vi "rszvl_core_global.vi"() -> ()   [LabVIEW 2014] (continued)
"Command"="DWEL"}]}, {"Name"="rszvl_rngNWASegmentRBW", "Type"=0, "Min?"=TRUE, "Max?"=TRUE, "Entries"=[{"Name"="", "Discrete or Min"=1e-06, "Max"=5000000.0, "Coerced"=0.0, "Command"=""}]}, {"Name"="rszvl_rngNWASegmentSelectivity", "Type"=2, "Min?"=FALSE, "Max?"=FALSE, "Entries"=[{"Name"="RSZVL_VAL_SEG_SELECTIVITY_NORMAL", "Discrete or Min"=0.0, "Max"=0.0, "Coerced"=0.0, "Command"="NORM"}, {"Name"="RSZVL_VAL_SEG_SELECTIVITY_FAST", "Discrete or Min"=1.0, "Max"=0.0, "Coerced"=0.0, "Command"="FAST"}]}, {"Name"="rszvl_rngNWASegmentSweepTime", "Type"=0, "Min?"=TRUE, "Max?"=TRUE, "Entries"=[{"Name"="", "Discrete or Min"=0.0, "Max"=1000.0, "Coerced"=0.0, "Command"=""}]}, {"Name"="rszvl_rngNWASegmentMeasDelay", "Type"=0, "Min?"=TRUE, "Max?"=TRUE, "Entries"=[{"Name"="", "Discrete or Min"=0.0, "Max"=2500.0, "Coerced"=0.0, "Command"=""}]}, {"Name"="rszvl_rngNWASegmentSweepPoints", "Type"=0, "Min?"=TRUE, "Max?"=TRUE, "Entries"=[{"Name"="", "Discrete or Min"=1.0, "Max"=4001.0, "Coerced"=0.0, "Command"=""}]}, {"Name"="rszvl_rngNWAConnectorType", "Type"=2, "Min?"=FALSE, "Max?"=FALSE, "Entries"=[{"Name"="RSZVL_VAL_CONN_N50FEMALE", "Discrete or Min"=0.0, "Max"=0.0, "Coerced"=0.0, "Command"="N50FEMALE"}, {"Name"="RSZVL_VAL_CONN_N50MALE", "Discrete or Min"=1.0, "Max"=0.0, "Coerced"=0.0, "Command"="N50MALE"}, {"Name"="RSZVL_VAL_CONN_N75FEMALE", "Discrete or Min"=2.0, "Max"=0.0, "Coerced"=0.0, "Command"="N75FEMALE"}, {"Name"="RSZVL_VAL_CONN_N75MALE", "Discrete or Min"=3.0, "Max"=0.0, "Coerced"=0.0, "Command"="N75MALE"}, {"Name"="RSZVL_VAL_CONN_PC7", "Discrete or Min"=4.0, "Max"=0.0, "Coerced"=0.0, "Command"="PC7"}, {"Name"="RSZVL_VAL_CONN_PC35FEMALE", "Discrete or Min"=5.0, "Max"=0.0, "Coerced"=0.0, "Command"="PC35FEMALE"}, {"Name"="RSZVL_VAL_CONN_PC35MALE", "Discrete or Min"=6.0, "Max"=0.0, "Coerced"=0.0, "Command"="PC35MALE"}, {"Name"="RSZVL_VAL_CONN_PC292FEMALE", "Discrete or Min"=7.0, "Max"=0.0, "Coerced"=0.0, "Command"="PC292FEMALE"}, {"Name"="RSZVL_VAL_CONN_PC292MALE", "Discrete or Min"=8.0, "Max"=0.0, "Coerced"=0.0, "Command"="PC292MALE"}, {"Name"="RSZVL_VAL_CONN_UFEMALE1", "Discrete or Min"=9.0, "Max"=0.0, "Coerced"=0.0, "Command"="UFEMALE1"}, {"Name"="RSZVL_VAL_CONN_UMALE1", "Discrete or Min"=10.0, "Max"=0.0, "Coerced"=0.0, "Command"="UMALE1"}, {"Name"="RSZVL_VAL_CONN_UFEMALE2", "Discrete or Min"=11.0, "Max"=0.0, "Coerced"=0.0, "Command"="UFEMALE2"}, {"Name"="RSZVL_VAL_CONN_UMALE2", "Discrete or Min"=12.0, "Max"=0.0, "Coerced"=0.0, "Command"="UMALE2"}]}, {"Name"="rszvl_rngNWASameConnectorsAtPorts", "Type"=2, "Min?"=FALSE, "Max?"=FALSE, "Entries"=[{"Name"="RSZVL_VAL_CONN_PORTS_SINGLE", "Discrete or Min"=0.0, "Max"=0.0, "Coerced"=0.0, "Command"="SING"}, {"Name"="RSZVL_VAL_CONN_PORTS_ALL", "Discrete or Min"=1.0, "Max"=0.0, "Coerced"=0.0, "Command"="ALL"}]}, {"Name"="rszvl_rngNWAOffsetLoss", "Type"=0, "Min?"=TRUE, "Max?"=TRUE, "Entries"=[{"Name"="", "Discrete or Min"=-200.0, "Max"=200.0, "Coerced"=0.0, "Command"=""}]}, {"Name"="rszvl_rngNWASourcePower", "Type"=0, "Min?"=TRUE, "Max?"=TRUE, "Entries"=[{"Name"="", "Discrete or Min"=-300.0, "Max"=20.0, "Coerced"=0.0, "Command"=""}]}, {"Name"="rszvl_rngNWATraceXOffset", "Type"=0, "Min?"=TRUE, "Max?"=TRUE, "Entries"=[{"Name"="", "Discrete or Min"=-999000000000.0, "Max"=999000000000.0, "Coerced"=0.0, "Command"=""}]}, {"Name"="rszvl_rngNWATraceFormat", "Type"=2, "Min?"=FALSE, "Max?"=FALSE, "Entries"=[{"Name"="RSZVL_VAL_TRAC_FORM_MLIN", "Discrete or Min"=0.0, "Max"=0.0, "Coerced"=0.0, "Command"="MLIN"}, {"Name"="RSZVL_VAL_TRAC_FORM_MLOG", "Discrete or Min"=1.0, "Max"=0.0, "Coerced"=0.0, "Command"="MLOG"}, {"Name"="RSZVL_VAL_TRAC_FORM_PHAS", "Discrete or Min"=2.0, "Max"=0.0, "Coerced"=0.0, "Command"="PHAS"}, {"Name"="RSZVL_VAL_TRAC_FORM_UPH", "Discrete or Min"=3.0, "Max"=0.0, "Coerced"=0.0, "Command"="UPH"}, {"Name"="RSZVL_VAL_TRAC_FORM_POL", "Discrete or Min"=4.0, "Max"=0.0, "Coerced"=0.0, "Command"="POL"}, {"Name"="RSZVL_VAL_TRAC_FORM_SMIT", "Discrete or Min"=5.0, "Max"=0.0, "Coerced"=0.0, "Command"="SMIT"}, {"Name"="RSZVL_VAL_TRAC_FORM_ISM", "Discrete or Min"=6.0, "Max"=0.0, "Coerced"=0.0, "Command"="ISM"}, {"Name"="RSZVL_VAL_TRAC_FORM_GDEL", "Discrete or Min"=7.0, "Max"=0.0, "Coerced"=0.0, "Command"="GDEL"}, {"Name"="RSZVL_VAL_TRAC_FORM_REAL", "Discrete or Min"=8.0, "Max"=0.0, "Coerced"=0.0, "Command"="REAL"}, {"Name"="RSZVL_VAL_TRAC_FORM_IMAG", "Discrete or Min"=9.0, "Max"=0.0, "Coerced"=0.0, "Command"="IMAG"}, {"Name"="RSZVL_VAL_TRAC_FORM_SWR", "Discrete or Min"=10.0, "Max"=0.0, "Coerced"=0.0, "Command"="SWR"}]}, {"Name"="rszvl_rngNWATraceMathFunction", "Type"=2, "Min?"=FALSE, "Max?"=FALSE, "Entries"=[{"Name"="RSZVL_VAL_TRAC_MATH_FUNC_NORM", "Discrete or Min"=0.0, "Max"=0.0, "Coerced"=0.0, "Command"="NORM"}, {"Name"="RSZVL_VAL_TRAC_MATH_FUNC_SUBT", "Discrete or Min"=1.0, "Max"=0.0, "Coerced"=0.0, "Command"="SUBT"}, {"Name"="RSZVL_VAL_TRAC_MATH_FUNC_DIV", "Discrete or Min"=2.0, "Max"=0.0, "Coerced"=0.0, "Command"="DIV"}]}, {"Name"="rszvl_rngNWATraceSmoothing", "Type"=0, "Min?"=TRUE, "Max?"=TRUE, "Entries"=[{"Name"="", "Discrete or Min"=0.05, "Max"=100.0, "Coerced"=0.0, "Command"=""}]}, {"Name"="rszvl_rngNWATraceMaxHold", "Type"=2, "Min?"=FALSE, "Max?"=FALSE, "Entries"=[{"Name"="RSZVL_VAL_TRAC_PHOL_OFF", "Discrete or Min"=0.0, "Max"=0.0, "Coerced"=0.0, "Command"="OFF"}, {"Name"="RSZVL_VAL_TRAC_PHOL_MAX", "Discrete or Min"=1.0, "Max"=0.0, "Coerced"=0.0, "Command"="MAX"}]}, {"Name"="rszvl_rngNWADeleteMemTrace", "Type"=2, "Min?"=FALSE, "Max?"=FALSE, "Entries"=[{"Name"="RSZVL_VAL_TRAC_DELETE_MDAT1", "Discrete or Min"=0.0, "Max"=0.0, "Coerced"=0.0, "Command"="MDATA1"}, {"Name"="RSZVL_VAL_TRAC_DELETE_MDAT2", "Discrete or Min"=1.0, "Max"=0.0, "Coerced"=0.0, "Command"="MDATA2"}, {"Name"="RSZVL_VAL_TRAC_DELETE_MDAT3", "Discrete or Min"=2.0, "Max"=0.0, "Coerced"=0.0, "Command"="MDATA3"}, {"Name"="RSZVL_VAL_TRAC_DELETE_MDAT4", "Discrete or Min"=3.0, "Max"=0.0, "Coerced"=0.0, "Command"="MDATA4"}, {"Name"="RSZVL_VAL_TRAC_DELETE_MDAT5", "Discrete or Min"=4.0, "Max"=0.0, "Coerced"=0.0, "Command"="MDATA5"}, {"Name"="RSZVL_VAL_TRAC_DELETE_MDAT6", "Discrete or Min"=5.0, "Max"=0.0, "Coerced"=0.0, "Command"="MDATA6"}, {"Name"="RSZVL_VAL_TRAC_DELETE_MDAT7", "Discrete or Min"=6.0, "Max"=0.0, "Coerced"=0.0, "Command"="MDATA7"}, {"Name"="RSZVL_VAL_TRAC_DELETE_MDAT8", "Discrete or Min"=7.0, "Max"=0.0, "Coerced"=0.0, "Command"="MDATA8"}]}, {"Name"="rszvl_rngNWATraceEvalRange", "Type"=2, "Min?"=FALSE, "Max?"=FALSE, "Entries"=[{"Name"="RSZVL_VAL_TRAC_EVAL_FULL_SPAN", "Discrete or Min"=0.0, "Max"=0.0, "Coerced"=0.0, "Command"="0"}, {"Name"="RSZVL_VAL_TRAC_EVAL_1", "Discrete or Min"=1.0, "Max"=0.0, "Coerced"=0.0, "Command"="1"}, {"Name"="RSZVL_VAL_TRAC_EVAL_2", "Discrete or Min"=2.0, "Max"=0.0, "Coerced"=0.0, "Command"="2"}, {"Name"="RSZVL_VAL_TRAC_EVAL_3", "Discrete or Min"=3.0, "Max"=0.0, "Coerced"=0.0, "Command"="3"}, {"Name"="RSZVL_VAL_TRAC_EVAL_4", "Discrete or Min"=4.0, "Max"=0.0, "Coerced"=0.0, "Command"="4"}, {"Name"="RSZVL_VAL_TRAC_EVAL_5", "Discrete or Min"=5.0, "Max"=0.0, "Coerced"=0.0, "Command"="5"}, {"Name"="RSZVL_VAL_TRAC_EVAL_6", "Discrete or Min"=6.0, "Max"=0.0, "Coerced"=0.0, "Command"="6"}, {"Name"="RSZVL_VAL_TRAC_EVAL_7", "Discrete or Min"=7.0, "Max"=0.0, "Coerced"=0.0, "Command"="7"}, {"Name"="RSZVL_VAL_TRAC_EVAL_8", "Discrete or Min"=8.0, "Max"=0.0, "Coerced"=0.0, "Command"="8"}, {"Name"="RSZVL_VAL_TRAC_EVAL_9", "Discrete or Min"=9.0, "Max"=0.0, "Coerced"=0.0, "Command"="9"}, {"Name"="RSZVL_VAL_TRAC_EVAL_10", "Discrete or Min"=10.0, "Max"=0.0, "Coerced"=0.0, "Command"="10"}]}, {"Name"="rszvl_rngNWATraceEvalRangeStart", "Type"=0, "Min?"=TRUE, "Max?"=TRUE, "Entries"=[{"Name"="", "Discrete or Min"=-1000000000000.0, "Max"=999999999999.0, "Coerced"=0.0, "Command"=""}]}, {"Name"="rszvl_rngNWATraceEvalRangeStop", "Type"=0, "Min?"=TRUE, "Max?"=TRUE, "Entries"=[{"Name"="", "Discrete or Min"=-999999999999.0, "Max"=1000000000000.0, "Coerced"=0.0, "Command"=""}]}, {"Name"="rszvl_rngNWAMarkerStimulus", "Type"=0, "Min?"=TRUE, "Max?"=TRUE, "Entries"=[{"Name"="", "Discrete or Min"=-990000000000.0, "Max"=990000000000.0, "Coerced"=0.0, "Command"=""}]}, {"Name"="rszvl_rngNWAMarkerMode", "Type"=2, "Min?"=FALSE, "Max?"=FALSE, "Entries"=[{"Name"="RSZVL_VAL_MARK_MODE_CONT", "Discrete or Min"=0.0, "Max"=0.0, "Coerced"=0.0, "Command"="CONT"}, {"Name"="RSZVL_VAL_MARK_MODE_DISC", "Discrete or Min"=1.0, "Max"=0.0, "Coerced"=0.0, "Command"="DISC"}]}, {"Name"="rszvl_rngNWAMarkerType", "Type"=2, "Min?"=FALSE, "Max?"=FALSE, "Entries"=[{"Name"="RSZVL_VAL_MARKER_TYPE_NORM", "Discrete or Min"=0.0, "Max"=0.0, "Coerced"=0.0, "Command"="NORM"}, {"Name"="RSZVL_VAL_MARKER_TYPE_FIX", "Discrete or Min"=1.0, "Max"=0.0, "Coerced"=0.0, "Command"="FIX"}]}, {"Name"="rszvl_rngNWAMarkerFormat", "Type"=2, "Min?"=FALSE, "Max?"=FALSE, "Entries"=[{"Name"="RSZVL_VAL_MARK_FORM_MLIN", "Discrete or Min"=0.0, "Max"=0.0, "Coerced"=0.0, "Command"="MLIN"}, {"Name"="RSZVL_VAL_MARK_FORM_MLOG", "Discrete or Min"=1.0, "Max"=0.0, "Coerced"=0.0, "Command"="MLOG"}, {"Name"="RSZVL_VAL_MARK_FORM_PHAS", "Discrete or Min"=2.0, "Max"=0.0, "Coerced"=0.0, "Command"="PHAS"}, {"Name"="RSZVL_VAL_MARK_FORM_POL", "Discrete or Min"=3.0, "Max"=0.0, "Coerced"=0.0, "Command"="POL"}, {"Name"="RSZVL_VAL_MARK_FORM_GDEL", "Discrete or Min"=4.0, "Max"=0.0, "Coerced"=0.0, "Command"="GDEL"}, {"Name"="RSZVL_VAL_MARK_FORM_REAL", "Discrete or Min"=5.0, "Max"=0.0, "Coerced"=0.0, "Command"="REAL"}, {"Name"="RSZVL_VAL_MARK_FORM_IMAG", "Discrete or Min"=6.0, "Max"=0.0, "Coerced"=0.0, "Command"="IMAG"}, {"Name"="RSZVL_VAL_MARK_FORM_SWR", "Discrete or Min"=7.0, "Max"=0.0, "Coerced"=0.0, "Command"="SWR"}, {"Name"="RSZVL_VAL_MARK_FORM_LINP", "Discrete or Min"=8.0, "Max"=0.0, "Coerced"=0.0, "Command"="LINP"}, {"Name"="RSZVL_VAL_MARK_FORM_LOGP", "Discrete or Min"=9.0, "Max"=0.0, "Coerced"=0.0, "Command"="LOGP"}, {"Name"="RSZVL_VAL_MARK_FORM_IMP", "Discrete or Min"=10.0, "Max"=0.0, "Coerced"=0.0, "Command"="IMP"}, {"Name"="RSZVL_VAL_MARK_FORM_ADM", "Discrete or Min"=11.0, "Max"=0.0, "Coerced"=0.0, "Command"="ADM"}]}, {"Name"="rszvl_rngNWAMarkerSearch", "Type"=2, "Min?"=FALSE, "Max?"=FALSE, "Entries"=[{"Name"="RSZVL_VAL_MARK_SEARCH_MAX", "Discrete or Min"=0.0, "Max"=0.0, "Coerced"=0.0, "Command"="MAX"}, {"Name"="RSZVL_VAL_MARK_SEARCH_MIN", "Discrete or Min"=1.0, "Max"=0.0, "Coerced"=0.0, "Command"="MIN"}, {"Name"="RSZVL_VAL_MARK_SEARCH_RPE", "Discrete or Min"=2.0, "Max"=0.0, "Coerced"=0.0, "Command"="RPE"}, {"Name"="RSZVL_VAL_MARK_SEARCH_LPE", "Discrete or Min"=3.0, "Max"=0.0, "Coerced"=0.0, "Command"="LPE"}, {"Name"="RSZVL_VAL_MARK_SEARCH_NPE", "Discrete or Min"=4.0, "Max"=0.0, "Coerced"=0.0, "Command"="NPE"}, {"Name"="RSZVL_VAL_MARK_SEARCH_TARG", "Discrete or Min"=5.0, "Max"=0.0, "Coerced"=0.0, "Command"="TARG"}, {"Name"="RSZVL_VAL_MARK_SEARCH_LTAR", "Discrete or Min"=6.0, "Max"=0.0, "Coerced"=0.0, "Command"="LTAR"}, {"Name"="RSZVL_VAL_MARK_SEARCH_RTAR", "Discrete or Min"=7.0, "Max"=0.0, "Coerced"=0.0, "Command"="RTAR"}, {"Name"="RSZVL_VAL_MARK_SEARCH_BFIL", "Discrete or Min"=8.0, "Max"=0.0, "Coerced"=0.0, "Command"="BFIL"}]}, {"Name"="rszvl_rngNWAMarkerBFilterSearchMode", "Type"=2, "Min?"=FALSE, "Max?"=FALSE, "Entries"=[{"Name"="RSZVL_VAL_MARK_BFIL_SEARCH_BPAS", "Discrete or Min"=0.0, "Max"=0.0, "Coerced"=0.0, "Command"="BPAS"}, {"Name"="RSZVL_VAL_MARK_BFIL_SEARCH_BST", "Discrete or Min"=1.0, "Max"=0.0, "Coerced"=0.0, "Command"="BST"}, {"Name"="RSZVL_VAL_MARK_BFIL_SEARCH_BPRM", "Discrete or Min"=2.0, "Max"=0.0, "Coerced"=0.0, "Command"="BPRM"}, {"Name"="RSZVL_VAL_MARK_BFIL_SEARCH_BSRM", "Discrete or Min"=3.0, "Max"=0.0, "Coerced"=0.0, "Command"="BSRM"}]}, {"Name"="rszvl_rngNWAMarkerSearchRange", "Type"=2, "Min?"=FALSE, "Max?"=FALSE, "Entries"=[{"Name"="RSZVL_VAL_MARK_FULL_SPAN", "Discrete or Min"=0.0, "Max"=0.0, "Coerced"=0.0, "Command"="0"}, {"Name"="RSZVL_VAL_MARK_RANGE_1", "Discrete or Min"=1.0, "Max"=0.0, "Coerced"=0.0, "Command"="1"}, {"Name"="RSZVL_VAL_MARK_RANGE_2", "Discrete or Min"=2.0, "Max"=0.0, "Coerced"=0.0, "Command"="2"}, {"Name"="RSZVL_VAL_MARK_RANGE_3", "Discrete or Min"=3.0, "Max"=0.0, "Coerced"=0.0, "Command"="3"}, {"Name"="RSZVL_VAL_MARK_RANGE_4", "Discrete or Min"=4.0, "Max"=0.0, "Coerced"=0.0, "Command"="4"}, {"Name"="RSZVL_VAL_MARK_RANGE_5", "Discrete or Min"=5.0, "Max"=0.0, "Coerced"=0.0, "Command"="5"}, {"Name"="RSZVL_VAL_MARK_RANGE_6", "Discrete or Min"=6.0, "Max"=0.0, "Coerced"=0.0, "Command"="6"}, {"Name"="RSZVL_VAL_MARK_RANGE_7", "Discrete or Min"=7.0, "Max"=0.0, "Coerced"=0.0, "Command"="7"}, {"Name"="RSZVL_VAL_MARK_RANGE_8", "Discrete or Min"=8.0, "Max"=0.0, "Coerced"=0.0, "Command"="8"}, {"Name"="RSZVL_VAL_MARK_RANGE_9", "Discrete or Min"=9.0, "Max"=0.0, "Coerced"=0.0, "Command"="9"}, {"Name"="RSZVL_VAL_MARK_RANGE_10", "Discrete or Min"=10.0, "Max"=0.0, "Coerced"=0.0, "Command"="10"}]}, {"Name"="rszvl_rngNWALimitRDOMComplex", "Type"=2, "Min?"=FALSE, "Max?"=FALSE, "Entries"=[{"Name"="RSZVL_VAL_LIM_RDOM_COMP_S", "Discrete or Min"=0.0, "Max"=0.0, "Coerced"=0.0, "Command"="S"}, {"Name"="RSZVL_VAL_LIM_RDOM_COMP_SINV", "Discrete or Min"=1.0, "Max"=0.0, "Coerced"=0.0, "Command"="SINV"}, {"Name"="RSZVL_VAL_LIM_RDOM_COMP_Y", "Discrete or Min"=2.0, "Max"=0.0, "Coerced"=0.0, "Command"="Y"}, {"Name"="RSZVL_VAL_LIM_RDOM_COMP_Z", "Discrete or Min"=3.0, "Max"=0.0, "Coerced"=0.0, "Command"="Z"}, {"Name"="RSZVL_VAL_LIM_RDOM_COMP_YREL", "Discrete or Min"=4.0, "Max"=0.0, "Coerced"=0.0, "Command"="YREL"}, {"Name"="RSZVL_VAL_LIM_RDOM_COMP_ZREL", "Discrete or Min"=5.0, "Max"=0.0, "Coerced"=0.0, "Command"="ZREL"}]}, {"Name"="rszvl_rngNWALimitRDOMFormat", "Type"=2, "Min?"=FALSE, "Max?"=FALSE, "Entries"=[{"Name"="RSZVL_VAL_LIM_RDOM_FORM_COMP", "Discrete or Min"=0.0, "Max"=0.0, "Coerced"=0.0, "Command"="COMP"}, {"Name"="RSZVL_VAL_LIM_RDOM_FORM_MAGN", "Discrete or Min"=1.0, "Max"=0.0, "Coerced"=0.0, "Command"="MAGN"}, {"Name"="RSZVL_VAL_LIM_RDOM_FORM_PHAS", "Discrete or Min"=2.0, "Max"=0.0, "Coerced"=0.0, "Command"="PHAS"}, {"Name"="RSZVL_VAL_LIM_RDOM_FORM_REAL", "Discrete or Min"=3.0, "Max"=0.0, "Coerced"=0.0, "Command"="REAL"}, {"Name"="RSZVL_VAL_LIM_RDOM_FORM_IMAG", "Discrete or Min"=4.0, "Max"=0.0, "Coerced"=0.0, "Command"="IMAG"}, {"Name"="RSZVL_VAL_LIM_RDOM_FORM_SWR", "Discrete or Min"=5.0, "Max"=0.0, "Coerced"=0.0, "Command"="SWR"}, {"Name"="RSZVL_VAL_LIM_RDOM_FORM_GDEL", "Discrete or Min"=6.0, "Max"=0.0, "Coerced"=0.0, "Command"="GDEL"}, {"Name"="RSZVL_VAL_LIM_RDOM_FORM_L", "Discrete or Min"=7.0, "Max"=0.0, "Coerced"=0.0, "Command"="L"}, {"Name"="RSZVL_VAL_LIM_RDOM_FORM_C", "Discrete or Min"=8.0, "Max"=0.0, "Coerced"=0.0, "Command"="C"}]}, {"Name"="rszvl_rngNWALimitRDOMSpacing", "Type"=2, "Min?"=FALSE, "Max?"=FALSE, "Entries"=[{"Name"="RSZVL_VAL_LIM_RDOM_SPAC_LIN", "Discrete or Min"=0.0, "Max"=0.0, "Coerced"=0.0, "Command"="LIN"}, {"Name"="RSZVL_VAL_LIM_RDOM_SPAC_LOG", "Discrete or Min"=1.0, "Max"=0.0, "Coerced"=0.0, "Command"="LOG"}, {"Name"="RSZVL_VAL_LIM_RDOM_SPAC_DB", "Discrete or Min"=2.0, "Max"=0.0, "Coerced"=0.0, "Command"="DB"}, {"Name"="RSZVL_VAL_LIM_RDOM_SPAC_SIC", "Discrete or Min"=3.0, "Max"=0.0, "Coerced"=0.0, "Command"="SIC"}]}, {"Name"="rszvl_rngNWALimitSegmType", "Type"=2, "Min?"=FALSE, "Max?"=FALSE, "Entries"=[{"Name"="RSZVL_VAL_LIMIT_OFF", "Discrete or Min"=0.0, "Max"=0.0, "Coerced"=0.0, "Command"="OFF"}, {"Name"="RSZVL_VAL_LIMIT_UPPER", "Discrete or Min"=1.0, "Max"=0.0, "Coerced"=0.0, "Command"="LMAX"}, {"Name"="RSZVL_VAL_LIMIT_LOWER", "Discrete or Min"=2.0, "Max"=0.0, "Coerced"=0.0, "Command"="LMIN"}]}, {"Name"="rszvl_rngNWAParamConversion", "Type"=2, "Min?"=FALSE, "Max?"=FALSE, "Entries"=[{"Name"="RSZVL_VAL_CONV_S", "Discrete or Min"=0.0, "Max"=0.0, "Coerced"=0.0, "Command"="S"}, {"Name"="RSZVL_VAL_CONV_Y", "Discrete or Min"=1.0, "Max"=0.0, "Coerced"=0.0, "Command"="Y"}, {"Name"="RSZVL_VAL_CONV_Z", "Discrete or Min"=2.0, "Max"=0.0, "Coerced"=0.0, "Command"="Z"}]}, {"Name"="rszvl_rngNWAColorScheme", "Type"=2, "Min?"=FALSE, "Max?"=FALSE, "Entries"=[{"Name"="RSZVL_VAL_COLOR_DBACKGROUND", "Discrete or Min"=0.0, "Max"=0.0, "Coerced"=0.0, "Command"="DBAC"}, {"Name"="RSZVL_VAL_COLOR_LBACKGROUND", "Discrete or Min"=1.0, "Max"=0.0, "Coerced"=0.0, "Command"="LBAC"}, {"Name"="RSZVL_VAL_COLOR_BW_LSTYLES", "Discrete or Min"=2.0, "Max"=0.0, "Coerced"=0.0, "Command"="BWLS"}, {"Name"="RSZVL_VAL_COLOR_BW_SOLID", "Discrete or Min"=3.0, "Max"=0.0, "Coerced"=0.0, "Command"="BWS"}]}, {"Name"="rszvl_rngNWAPresetScope", "Type"=2, "Min?"=FALSE, "Max?"=FALSE, "Entries"=[{"Name"="RSZVL_VAL_PRESET_SINGLE", "Discrete or Min"=0.0, "Max"=0.0, "Coerced"=0.0, "Command"="SING"}, {"Name"="RSZVL_VAL_PRESET_ALL", "Discrete or Min"=1.0, "Max"=0.0, "Coerced"=0.0, "Command"="ALL"}]}, {"Name"="rszvl_rngInstrMode", "Type"=2, "Min?"=FALSE, "Max?"=FALSE, "Entries"=[{"Name"="RSZVL_VAL_SAN", "Discrete or Min"=0.0, "Max"=0.0, "Coerced"=0.0, "Command"="SAN"}, {"Name"="RSZVL_VAL_NWA", "Discrete or Min"=1.0, "Max"=0.0, "Coerced"=0.0, "Command"="NWA"}, {"Name"="RSZVL_VAL_NOISE", "Discrete or Min"=2.0, "Max"=0.0, "Coerced"=0.0, "Command"="NOIS"}, {"Name"="RSZVL_VAL_BWCD", "Discrete or Min"=3.0, "Max"=0.0, "Coerced"=0.0, "Command"="BWCD"}, {"Name"="RSZVL_VAL_WLAN", "Discrete or Min"=4.0, "Max"=0.0, "Coerced"=0.0, "Command"="WLAN"}, {"Name"="RSZVL_VAL_WIMAX", "Discrete or Min"=5.0, "Max"=0.0, "Coerced"=0.0, "Command"="WIM"}, {"Name"="RSZVL_VAL_ADEM", "Discrete or Min"=6.0, "Max"=0.0, "Coerced"=0.0, "Command"="ADEM"}, {"Name"="RSZVL_VAL_BTO", "Discrete or Min"=7.0, "Max"=0.0, "Coerced"=0.0, "Command"="BTO"}, {"Name"="RSZVL_VAL_CATV", "Discrete or Min"=8.0, "Max"=0.0, "Coerced"=0.0, "Command"="CATV"}]}, {"Name"="rszvl_rngNWADFaultStart", "Type"=0, "Min?"=TRUE, "Max?"=TRUE, "Entries"=[{"Name"="", "Discrete or Min"=-5.0, "Max"=9.9999, "Coerced"=0.0, "Command"=""}]}, {"Name"="rszvl_rngNWADFaultStop", "Type"=0, "Min?"=TRUE, "Max?"=TRUE, "Entries"=[{"Name"="", "Discrete or Min"=-4.999, "Max"=10.0, "Coerced"=0.0, "Command"=""}]}, {"Name"="rszvl_rngNWADFaultSpan", "Type"=0, "Min?"=TRUE, "Max?"=TRUE, "Entries"=[{"Name"="", "Discrete or Min"=0.001, "Max"=15.0, "Coerced"=0.0, "Command"=""}]}, {"Name"="rszvl_rngNWASegmentAtten", "Type"=0, "Min?"=TRUE, "Max?"=TRUE, "Entries"=[{"Name"="", "Discrete or Min"=0.0, "Max"=30.0, "Coerced"=0.0, "Command"=""}]}, {"Name"="rszvl_rngNWASegmentPower", "Type"=0, "Min?"=TRUE, "Max?"=TRUE, "Entries"=[{"Name"="", "Discrete or Min"=-40.0, "Max"=10.0, "Coerced"=0.0, "Command"=""}]}, {"Name"="rszvl_rngHcopyPageSettings", "Type"=2, "Min?"=FALSE, "Max?"=FALSE, "Entries"=[{"Name"="RSZVL_VAL_HCOPY_ACT", "Discrete or Min"=0.0, "Max"=0.0, "Coerced"=0.0, "Command"="ACT"}, {"Name"="RSZVL_VAL_HCOPY_ALL", "Discrete or Min"=1.0, "Max"=0.0, "Coerced"=0.0, "Command"="ALL"}, {"Name"="RSZVL_VAL_HCOPY_SING", "Discrete or Min"=2.0, "Max"=0.0, "Coerced"=0.0, "Command"="SING"}]}, {"Name"="rszvl_rngNWAGetCalState", "Type"=2, "Min?"=FALSE, "Max?"=FALSE, "Entries"=[{"Name"="RSZVL_CALSTATE_CAL", "Discrete or Min"=0.0, "Max"=0.0, "Coerced"=0.0, "Command"="CAL"}, {"Name"="RSZVL_CALSTATE_CAI", "Discrete or Min"=1.0, "Max"=0.0, "Coerced"=0.0, "Command"="CAI"}, {"Name"="RSZVL_CALSTATE_CA", "Discrete or Min"=2.0, "Max"=0.0, "Coerced"=0.0, "Command"="CA?"}, {"Name"="RSZVL_CALSTATE_CAV", "Discrete or Min"=3.0, "Max"=0.0, "Coerced"=0.0, "Command"="CAV"}, {"Name"="RSZVL_CALSTATE_CALOFF", "Discrete or Min"=4.0, "Max"=0.0, "Coerced"=0.0, "Command"="CAL OFF"}]}, {"Name"="rszvl_rngFmTriggerSource", "Type"=2, "Min?"=FALSE, "Max?"=FALSE, "Entries"=[{"Name"="RSZVL_VAL_TRG_IMM", "Discrete or Min"=0.0, "Max"=0.0, "Coerced"=0.0, "Command"="IMM"}, {"Name"="RSZVL_VAL_TRG_EXT", "Discrete or Min"=1.0, "Max"=0.0, "Coerced"=0.0, "Command"="EXT"}, {"Name"="RSZVL_VAL_TRG_IFP", "Discrete or Min"=2.0, "Max"=0.0, "Coerced"=0.0, "Command"="IFP"}, {"Name"="RSZVL_VAL_TRG_FM", "Discrete or Min"=3.0, "Max"=0.0, "Coerced"=0.0, "Command"="FM"}, {"Name"="RSZVL_VAL_TRG_AM", "Discrete or Min"=4.0, "Max"=0.0, "Coerced"=0.0, "Command"="AM"}, {"Name"="RSZVL_VAL_TRG_PM", "Discrete or Min"=5.0, "Max"=0.0, "Coerced"=0.0, "Command"="PM"}, {"Name"="RSZVL_VAL_TRG_AMR", "Discrete or Min"=6.0, "Max"=0.0, "Coerced"=0.0, "Command"="AMR"}]}, {"Name"="rszvl_rngAdemTrigAMLevelAbs", "Type"=0, "Min?"=TRUE, "Max?"=TRUE, "Entries"=[{"Name"="", "Discrete or Min"=-100.0, "Max"=30.0, "Coerced"=0.0, "Command"=""}]}, {"Name"="rszvl_rngAdemTrigAMLevelRel", "Type"=0, "Min?"=TRUE, "Max?"=TRUE, "Entries"=[{"Name"="", "Discrete or Min"=-100.0, "Max"=100.0, "Coerced"=0.0, "Command"=""}]}, {"Name"="rszvl_rngAdemTrigFMLevel", "Type"=0, "Min?"=TRUE, "Max?"=TRUE, "Entries"=[{"Name"="", "Discrete or Min"=-10000000.0, "Max"=10000000.0, "Coerced"=0.0, "Command"=""}]}, {"Name"="rszvl_rngAdemTrigPMLevel", "Type"=0, "Min?"=TRUE, "Max?"=TRUE, "Entries"=[{"Name"="", "Discrete or Min"=-1000.0, "Max"=1000.0, "Coerced"=0.0, "Command"=""}]}, {"Name"="rszvl_rngCoupling", "Type"=2, "Min?"=FALSE, "Max?"=FALSE, "Entries"=[{"Name"="RSZVL_VAL_DC", "Discrete or Min"=0.0, "Max"=0.0, "Coerced"=0.0, "Command"="DC"}, {"Name"="RSZVL_VAL_AC", "Discrete or Min"=1.0, "Max"=0.0, "Coerced"=0.0, "Command"="AC"}]}, {"Name"="rszvl_rngFmBwid", "Type"=0, "Min?"=TRUE, "Max?"=TRUE, "Entries"=[{"Name"="", "Discrete or Min"=100.0, "Max"=50000000.0, "Coerced"=0.0, "Command"=""}]}, {"Name"="rszvl_rngAdemPhaseWrap", "Type"=2, "Min?"=FALSE, "Max?"=FALSE, "Entries"=[{"Name"="RSZVL_VAL_ADEM_UPHAS", "Discrete or Min"=0.0, "Max"=0.0, "Coerced"=0.0, "Command"="UPH"}, {"Name"="RSZVL_VAL_ADEM_PHAS", "Discrete or Min"=1.0, "Max"=0.0, "Coerced"=0.0, "Command"="PHAS"}]}, {"Name"="rszvl_rngUnitAngle", "Type"=2, "Min?"=FALSE, "Max?"=FALSE, "Entries"=[{"Name"="RSZVL_VAL_UNIT_ANGLE_DEG", "Discrete or Min"=0.0, "Max"=0.0, "Coerced"=0.0, "Command"="DEG"}, {"Name"="RSZVL_VAL_UNIT_ANGLE_RAD", "Discrete or Min"=1.0, "Max"=0.0, "Coerced"=0.0, "Command"="RAD"}]}, {"Name"="rszvl_rngAdemBandRes", "Type"=0, "Min?"=TRUE, "Max?"=TRUE, "Entries"=[{"Name"="", "Discrete or Min"=1.0, "Max"=10000000.0, "Coerced"=0.0, "Command"=""}]}, {"Name"="rszvl_rngHpasFilterFreq", "Type"=1, "Min?"=FALSE, "Max?"=FALSE, "Entries"=[{"Name"="", "Discrete or Min"=0.0, "Max"=0.0, "Coerced"=50.0, "Command"=""}, {"Name"="", "Discrete or Min"=0.0, "Max"=0.0, "Coerced"=300.0, "Command"=""}]}, {"Name"="rszvl_rngLpasFiltFreq", "Type"=1, "Min?"=FALSE, "Max?"=FALSE, "Entries"=[{"Name"="", "Discrete or Min"=0.0, "Max"=0.0, "Coerced"=3000.0, "Command"=""}, {"Name"="", "Discrete or Min"=0.0, "Max"=0.0, "Coerced"=15000.0, "Command"=""}, {"Name"="", "Discrete or Min"=0.0, "Max"=0.0, "Coerced"=150000.0, "Command"=""}]}, {"Name"="rszvl_rngFiltDempTimeConst", "Type"=1, "Min?"=FALSE, "Max?"=FALSE, "Entries"=[{"Name"="", "Discrete or Min"=0.0, "Max"=0.0, "Coerced"=2.5e-05, "Command"=""}, {"Name"="", "Discrete or Min"=0.0, "Max"=0.0, "Coerced"=5e-05, "Command"=""}, {"Name"="", "Discrete or Min"=0.0, "Max"=0.0, "Coerced"=7.5e-05, "Command"=""}, {"Name"="", "Discrete or Min"=0.0, "Max"=0.0, "Coerced"=0.00075, "Command"=""}]}, {"Name"="rszvl_rngFiltDempPctConst", "Type"=1, "Min?"=FALSE, "Max?"=FALSE, "Entries"=[{"Name"="", "Discrete or Min"=0.0, "Max"=0.0, "Coerced"=5.0, "Command"=""}, {"Name"="", "Discrete or Min"=0.0, "Max"=0.0, "Coerced"=10.0, "Command"=""}, {"Name"="", "Discrete or Min"=0.0, "Max"=0.0, "Coerced"=25.0, "Command"=""}]}, {"Name"="rszvl_rngBtoWritePtype", "Type"=2, "Min?"=FALSE, "Max?"=FALSE, "Entries"=[{"Name"="RSZVL_VAL_BTO_PTYPE_AUTO", "Discrete or Min"=0.0, "Max"=0.0, "Coerced"=0.0, "Command"="AUTO"}, {"Name"="RSZVL_VAL_BTO_PTYPE_DH1", "Discrete or Min"=1.0, "Max"=0.0, "Coerced"=0.0, "Command"="DH1"}, {"Name"="RSZVL_VAL_BTO_PTYPE_DH3", "Discrete or Min"=2.0, "Max"=0.0, "Coerced"=0.0, "Command"="DH3"}, {"Name"="RSZVL_VAL_BTO_PTYPE_DH5", "Discrete or Min"=3.0, "Max"=0.0, "Coerced"=0.0, "Command"="DH5"}]}, {"Name"="rszvl_rngBtoPrat", "Type"=1, "Min?"=FALSE, "Max?"=FALSE, "Entries"=[{"Name"="", "Discrete or Min"=0.0, "Max"=0.0, "Coerced"=2.0, "Command"=""}, {"Name"="", "Discrete or Min"=0.0, "Max"=0.0, "Coerced"=4.0, "Command"=""}, {"Name"="", "Discrete or Min"=0.0, "Max"=0.0, "Coerced"=8.0, "Command"=""}, {"Name"="", "Discrete or Min"=0.0, "Max"=0.0, "Coerced"=16.0, "Command"=""}, {"Name"="", "Discrete or Min"=0.0, "Max"=0.0, "Coerced"=32.0, "Command"=""}]}, {"Name"="rszvl_rngBtoPcl", "Type"=0, "Min?"=TRUE, "Max?"=TRUE, "Entries"=[{"Name"="", "Discrete or Min"=1.0, "Max"=3.0, "Coerced"=0.0, "Command"=""}]}, {"Name"="rszvl_rngBtoBwid", "Type"=0, "Min?"=TRUE, "Max?"=TRUE, "Entries"=[{"Name"="", "Discrete or Min"=300000.0, "Max"=10000000.0, "Coerced"=0.0, "Command"=""}]}, {"Name"="rszvl_rngBtoVideo", "Type"=0, "Min?"=TRUE, "Max?"=TRUE, "Entries"=[{"Name"="", "Discrete or Min"=1.0, "Max"=1000000.0, "Coerced"=0.0, "Command"=""}]}, {"Name"="rszvl_rngBtoMeasFilt", "Type"=2, "Min?"=FALSE, "Max?"=FALSE, "Entries"=[{"Name"="RSZVL_BTO_MEASFILT_OFF", "Discrete or Min"=0.0, "Max"=0.0, "Coerced"=0.0, "Command"="OFF"}, {"Name"="RSZVL_BTO_MEASFILT_BTO", "Discrete or Min"=1.0, "Max"=0.0, "Coerced"=0.0, "Command"="BTO"}]}, {"Name"="rszvl_rngTraceModeWithBlank", "Type"=2, "Min?"=FALSE, "Max?"=FALSE, "Entries"=[{"Name"="RSZVL_TRAC_MOD_WRITE", "Discrete or Min"=0.0, "Max"=0.0, "Coerced"=0.0, "Command"="WRIT"}, {"Name"="RSZVL_TRAC_MOD_VIEW", "Discrete or Min"=1.0, "Max"=0.0, "Coerced"=0.0, "Command"="VIEW"}, {"Name"="RSZVL_TRAC_MOD_AVER", "Discrete or Min"=2.0, "Max"=0.0, "Coerced"=0.0, "Command"="AVER"}, {"Name"="RSZVL_TRAC_MOD_MAXH", "Discrete or Min"=3.0, "Max"=0.0, "Coerced"=0.0, "Command"="MAXH"}, {"Name"="RSZVL_TRAC_MOD_MINH", "Discrete or Min"=4.0, "Max"=0.0, "Coerced"=0.0, "Command"="MINH"}, {"Name"="RSZVL_TRAC_MOD_BLANK", "Discrete or Min"=5.0, "Max"=0.0, "Coerced"=0.0, "Command"="BLAN"}]}, {"Name"="rszvl_rngBtoTraceDetector", "Type"=2, "Min?"=FALSE, "Max?"=FALSE, "Entries"=[{"Name"="RSZVL_BTO_TRAC_DET_APEAK", "Discrete or Min"=0.0, "Max"=0.0, "Coerced"=0.0, "Command"="APE"}, {"Name"="RSZVL_BTO_TRAC_DET_NEG", "Discrete or Min"=1.0, "Max"=0.0, "Coerced"=0.0, "Command"="NEG"}, {"Name"="RSZVL_BTO_TRAC_DET_POS", "Discrete or Min"=2.0, "Max"=0.0, "Coerced"=0.0, "Command"="POS"}, {"Name"="RSZVL_BTO_TRAC_DET_SAMPLE", "Discrete or Min"=3.0, "Max"=0.0, "Coerced"=0.0, "Command"="SAMP"}, {"Name"="RSZVL_BTO_TRAC_DET_RMS", "Discrete or Min"=4.0, "Max"=0.0, "Coerced"=0.0, "Command"="RMS"}, {"Name"="RSZVL_BTO_TRAC_DET_AVER", "Discrete or Min"=5.0, "Max"=0.0, "Coerced"=0.0, "Command"="AVER"}]}, {"Name"="rszvl_rngBtoMeasMode", "Type"=2, "Min?"=FALSE, "Max?"=FALSE, "Entries"=[{"Name"="RSZVL_BTO_MEAS_MODE_OPOW", "Discrete or Min"=0.0, "Max"=0.0, "Coerced"=0.0, "Command"="OPOW"}, {"Name"="RSZVL_BTO_MEAS_MODE_ACLR", "Discrete or Min"=1.0, "Max"=0.0, "Coerced"=0.0, "Command"="ACLR"}, {"Name"="RSZVL_BTO_MEAS_MODE_MCH", "Discrete or Min"=2.0, "Max"=0.0, "Coerced"=0.0, "Command"="MCH"}, {"Name"="RSZVL_BTO_MEAS_MODE_ICFT", "Discrete or Min"=3.0, "Max"=0.0, "Coerced"=0.0, "Command"="ICFT"}, {"Name"="RSZVL_BTO_MEAS_MODE_CFDR", "Discrete or Min"=4.0, "Max"=0.0, "Coerced"=0.0, "Command"="CFDR"}, {"Name"="RSZVL_BTO_MEAS_MODE_RTP", "Discrete or Min"=5.0, "Max"=0.0, "Coerced"=0.0, "Command"="RTP"}, {"Name"="RSZVL_BTO_MEAS_MODE_IBS", "Discrete or Min"=6.0, "Max"=0.0, "Coerced"=0.0, "Command"="IBS"}, {"Name"="RSZVL_BTO_MEAS_MODE_DPEN", "Discrete or Min"=7.0, "Max"=0.0, "Coerced"=0.0, "Command"="DPEN"}, {"Name"="RSZVL_BTO_MEAS_MODE_CFST", "Discrete or Min"=8.0, "Max"=0.0, "Coerced"=0.0, "Command"="CFST"}]}, {"Name"="rszvl_rngBtoAclrAcp", "Type"=0, "Min?"=TRUE, "Max?"=TRUE, "Entries"=[{"Name"="", "Discrete or Min"=1.0, "Max"=78.0, "Coerced"=0.0, "Command"=""}]}, {"Name"="rszvl_rngBtoAntennaGain", "Type"=0, "Min?"=TRUE, "Max?"=TRUE, "Entries"=[{"Name"="", "Discrete or Min"=-200.0, "Max"=200.0, "Coerced"=0.0, "Command"=""}]}, {"Name"="rszvl_rngBtoBurstOffs", "Type"=0, "Min?"=TRUE, "Max?"=TRUE, "Entries"=[{"Name"="", "Discrete or Min"=-0.01, "Max"=0.01, "Coerced"=0.0, "Command"=""}]}, {"Name"="rszvl_rngBtoSyncOffs", "Type"=0, "Min?"=TRUE, "Max?"=TRUE, "Entries"=[{"Name"="", "Discrete or Min"=-10000.0, "Max"=10000.0, "Coerced"=0.0, "Command"=""}]}, {"Name"="rszvl_rngBtoSearchTime", "Type"=0, "Min?"=TRUE, "Max?"=TRUE, "Entries"=[{"Name"="", "Discrete or Min"=0.0001, "Max"=0.06528, "Coerced"=0.0, "Command"=""}]}, {"Name"="rszvl_rngBtoCfstBlockCount", "Type"=0, "Min?"=TRUE, "Max?"=TRUE, "Entries"=[{"Name"="", "Discrete or Min"=0.0, "Max"=1000000.0, "Coerced"=0.0, "Command"=""}]}, {"Name"="rszvl_rngBtoPayloadBytes", "Type"=0, "Min?"=TRUE, "Max?"=TRUE, "Entries"=[{"Name"="", "Discrete or Min"=1.0, "Max"=1000.0, "Coerced"=0.0, "Command"=""}]}, {"Name"="rszvl_rngBtoPtype", "Type"=2, "Min?"=FALSE, "Max?"=FALSE, "Entries"=[{"Name"="RSZVL_VAL_BTO_PTYPE_AUTO", "Discrete or Min"=0.0, "Max"=0.0, "Coerced"=0.0, "Command"="AUTO"}, {"Name"="RSZVL_VAL_BTO_PTYPE_DH1", "Discrete or Min"=1.0, "Max"=0.0, "Coerced"=0.0, "Command"="DH1"}, {"Name"="RSZVL_VAL_BTO_PTYPE_DH3", "Discrete or Min"=2.0, "Max"=0.0, "Coerced"=0.0, "Command"="DH3"}, {"Name"="RSZVL_VAL_BTO_PTYPE_DH5", "Discrete or Min"=3.0, "Max"=0.0, "Coerced"=0.0, "Command"="DH5"}, {"Name"="RSZVL_BTO_PTYPE_DM1", "Discrete or Min"=4.0, "Max"=0.0, "Coerced"=0.0, "Command"="DM1"}, {"Name"="RSZVL_BTO_PTYPE_DM3", "Discrete or Min"=5.0, "Max"=0.0, "Coerced"=0.0, "Command"="DM3"}, {"Name"="RSZVL_BTO_PTYPE_DM5", "Discrete or Min"=6.0, "Max"=0.0, "Coerced"=0.0, "Command"="DM5"}, {"Name"="RSZVL_BTO_PTYPE_FHS", "Discrete or Min"=7.0, "Max"=0.0, "Coerced"=0.0, "Command"="FHS"}, {"Name"="RSZVL_BTO_PTYPE_HV1", "Discrete or Min"=8.0, "Max"=0.0, "Coerced"=0.0, "Command"="HV1"}, {"Name"="RSZVL_BTO_PTYPE_HV2", "Discrete or Min"=9.0, "Max"=0.0, "Coerced"=0.0, "Command"="HV2"}, {"Name"="RSZVL_BTO_PTYPE_HV3", "Discrete or Min"=10.0, "Max"=0.0, "Coerced"=0.0, "Command"="HV3"}, {"Name"="RSZVL_BTO_PTYPE_DV", "Discrete or Min"=11.0, "Max"=0.0, "Coerced"=0.0, "Command"="DV"}, {"Name"="RSZVL_BTO_PTYPE_NULL", "Discrete or Min"=12.0, "Max"=0.0, "Coerced"=0.0, "Command"="NULL"}, {"Name"="RSZVL_BTO_PTYPE_POLL", "Discrete or Min"=13.0, "Max"=0.0, "Coerced"=0.0, "Command"="POLL"}, {"Name"="RSZVL_BTO_PTYPE_AUX1", "Discrete or Min"=14.0, "Max"=0.0, "Coerced"=0.0, "Command"="AUX1"}, {"Name"="RSZVL_BTO_PTYPE_UNDEF", "Discrete or Min"=15.0, "Max"=0.0, "Coerced"=0.0, "Command"="UNDEF"}]}, {"Name"="rszvl_rngSpemColor", "Type"=2, "Min?"=FALSE, "Max?"=FALSE, "Entries"=[{"Name"="RSZVL_VAL_SPEM_COL_COLOR", "Discrete or Min"=0.0, "Max"=0.0, "Coerced"=0.0, "Command"="COL"}, {"Name"="RSZVL_VAL_SPEM_COL_RADAR", "Discrete or Min"=1.0, "Max"=0.0, "Coerced"=0.0, "Command"="RAD"}, {"Name"="RSZVL_VAL_SPEM_COL_GRAY", "Discrete or Min"=2.0, "Max"=0.0, "Coerced"=0.0, "Command"="GRAY"}]}, {"Name"="rszvl_rngSpemHistoryBuffDepth", "Type"=0, "Min?"=TRUE, "Max?"=TRUE, "Entries"=[{"Name"="", "Discrete or Min"=282.0, "Max"=20000.0, "Coerced"=0.0, "Command"=""}]}, {"Name"="rszvl_rngSpemSearchArea", "Type"=2, "Min?"=FALSE, "Max?"=FALSE, "Entries"=[{"Name"="RSZVL_VAL_SPEM_SAR_MEMORY", "Discrete or Min"=1.0, "Max"=0.0, "Coerced"=0.0, "Command"="MEM"}, {"Name"="RSZVL_VAL_SPEM_SAR_VISIBLE", "Discrete or Min"=0.0, "Max"=0.0, "Coerced"=0.0, "Command"="VIS"}]}, {"Name"="rszvl_rngNoiseCalcLimLine", "Type"=2, "Min?"=FALSE, "Max?"=FALSE, "Entries"=[{"Name"="RSZVL_VAL_NOISE_CALC_LIM_LINE_NFIGURE", "Discrete or Min"=0.0, "Max"=0.0, "Coerced"=0.0, "Command"="NFIG"}, {"Name"="RSZVL_VAL_NOISE_CALC_LIM_LINE_TEFFECTIVE", "Discrete or Min"=1.0, "Max"=0.0, "Coerced"=0.0, "Command"="TEFF"}, {"Name"="RSZVL_VAL_NOISE_CALC_LIM_LINE_GAIN", "Discrete or Min"=2.0, "Max"=0.0, "Coerced"=0.0, "Command"="GAIN"}]}, {"Name"="rszvl_rngNoiseERNModeSel", "Type"=2, "Min?"=FALSE, "Max?"=FALSE, "Entries"=[{"Name"="RSZVL_VAL_NOISE_ERN_MODE_SEL_TABLE", "Discrete or Min"=0.0, "Max"=0.0, "Coerced"=0.0, "Command"="TABL"}, {"Name"="RSZVL_VAL_NOISE_ERN_MODE_SEL_SPOT", "Discrete or Min"=1.0, "Max"=0.0, "Coerced"=0.0, "Command"="SPOT"}]}, {"Name"="rszvl_rngNoiseLossMode", "Type"=2, "Min?"=FALSE, "Max?"=FALSE, "Entries"=[{"Name"="RSZVL_VAL_NOISE_LOSS_MODE_TABLE", "Discrete or Min"=0.0, "Max"=0.0, "Coerced"=0.0, "Command"="TABL"}, {"Name"="RSZVL_VAL_NOISE_LOSS_MODE_SPOT", "Discrete or Min"=1.0, "Max"=0.0, "Coerced"=0.0, "Command"="SPOT"}]}, {"Name"="rszvl_rngNoiseConfDUT", "Type"=2, "Min?"=FALSE, "Max?"=FALSE, "Entries"=[{"Name"="RSZVL_VAL_NOISE_CONF_DUT_AMPLIFIER", "Discrete or Min"=0.0, "Max"=0.0, "Coerced"=0.0, "Command"="AMPL"}, {"Name"="RSZVL_VAL_NOISE_CONF_DUT_DOWNCONV", "Discrete or Min"=1.0, "Max"=0.0, "Coerced"=0.0, "Command"="DOWN"}, {"Name"="RSZVL_VAL_NOISE_CONF_DUT_UPCONV", "Discrete or Min"=2.0, "Max"=0.0, "Coerced"=0.0, "Command"="UPC"}]}, {"Name"="rszvl_rngNoiseGPIBGenAddr", "Type"=0, "Min?"=TRUE, "Max?"=TRUE, "Entries"=[{"Name"="", "Discrete or Min"=0.0, "Max"=30.0, "Coerced"=0.0, "Command"=""}]}, {"Name"="rszvl_rngNoiseDispDataTrac", "Type"=2, "Min?"=FALSE, "Max?"=FALSE, "Entries"=[{"Name"="RSZVL_VAL_NOISE_DISP_DATA_TEFF", "Discrete or Min"=1.0, "Max"=0.0, "Coerced"=0.0, "Command"="TEFF"}, {"Name"="RSZVL_VAL_NOISE_DISP_DATA_NFIGURE", "Discrete or Min"=2.0, "Max"=0.0, "Coerced"=0.0, "Command"="NFIG"}]}, {"Name"="rszvl_rngNoiseXAxisFrequency", "Type"=2, "Min?"=FALSE, "Max?"=FALSE, "Entries"=[{"Name"="RSZVL_VAL_NOISE_XAXIS_IF", "Discrete or Min"=0.0, "Max"=0.0, "Coerced"=0.0, "Command"="IF"}, {"Name"="RSZVL_VAL_NOISE_XAXIS_RF", "Discrete or Min"=1.0, "Max"=0.0, "Coerced"=0.0, "Command"="RF"}]}, {"Name"="rszvl_rng3GBSMeas", "Type"=2, "Min?"=FALSE, "Max?"=FALSE, "Entries"=[{"Name"="RSZVL_VAL_3GPPBS_MEAS_POW", "Discrete or Min"=0.0, "Max"=0.0, "Coerced"=0.0, "Command"="POW"}, {"Name"="RSZVL_VAL_3GPPBS_MEAS_ACLR", "Discrete or Min"=1.0, "Max"=0.0, "Coerced"=0.0, "Command"="ACLR"}, {"Name"="RSZVL_VAL_3GPPBS_MEAS_ESP", "Discrete or Min"=2.0, "Max"=0.0, "Coerced"=0.0, "Command"="ESP"}, {"Name"="RSZVL_VAL_3GPPBS_MEAS_WCDP", "Discrete or Min"=3.0, "Max"=0.0, "Coerced"=0.0, "Command"="WCDP"}]}, {"Name"="rszvl_rng3GBSSyncType", "Type"=2, "Min?"=FALSE, "Max?"=FALSE, "Entries"=[{"Name"="RSZVL_VAL_3GPP_BS_SETTINGS_SYNC_TYPE_CPIC", "Discrete or Min"=0.0, "Max"=0.0, "Coerced"=0.0, "Command"="CPIC"}, {"Name"="RSZVL_VAL_3GPP_BS_SETTINGS_SYNC_TYPE_SCH", "Discrete or Min"=1.0, "Max"=0.0, "Coerced"=0.0, "Command"="SCH"}]}, {"Name"="rszvl_rng3GBSPowRef", "Type"=2, "Min?"=FALSE, "Max?"=FALSE, "Entries"=[{"Name"="RSZVL_VAL_3GPP_BS_SETTINGS_POW_REF_TOT", "Discrete or Min"=0.0, "Max"=0.0, "Coerced"=0.0, "Command"="TOT"}, {"Name"="RSZVL_VAL_3GPP_BS_SETTINGS_POW_REF_CPIC", "Discrete or Min"=1.0, "Max"=0.0, "Coerced"=0.0, "Command"="CPIC"}]}, {"Name"="rszvl_rng3GPPThr", "Type"=0, "Min?"=TRUE, "Max?"=TRUE, "Entries"=[{"Name"="", "Discrete or Min"=-100.0, "Max"=10.0, "Coerced"=0.0, "Command"=""}]}, {"Name"="rszvl_rng3GBSAntenna", "Type"=2, "Min?"=FALSE, "Max?"=FALSE, "Entries"=[{"Name"="RSZVL_VAL_3GPP_BS_SETTINGS_ANTENNA_OFF", "Discrete or Min"=0.0, "Max"=0.0, "Coerced"=0.0, "Command"="OFF"}, {"Name"="RSZVL_VAL_3GPP_BS_SETTINGS_ANTENNA_1", "Discrete or Min"=1.0, "Max"=0.0, "Coerced"=0.0, "Command"="1"}, {"Name"="RSZVL_VAL_3GPP_BS_SETTINGS_ANTENNA_2", "Discrete or Min"=2.0, "Max"=0.0, "Coerced"=0.0, "Command"="2"}]}, {"Name"="rszvl_rng3GUECDPScrCode", "Type"=0, "Min?"=TRUE, "Max?"=TRUE, "Entries"=[{"Name"="", "Discrete or Min"=0.0, "Max"=24575.0, "Coerced"=0.0, "Command"=""}]}, {"Name"="rszvl_rng3GBSChannel", "Type"=0, "Min?"=TRUE, "Max?"=TRUE, "Entries"=[{"Name"="", "Discrete or Min"=0.0, "Max"=511.0, "Coerced"=0.0, "Command"=""}]}, {"Name"="rszvl_rng3GPPSlotNum", "Type"=0, "Min?"=TRUE, "Max?"=TRUE, "Entries"=[{"Name"="", "Discrete or Min"=0.0, "Max"=14.0, "Coerced"=0.0, "Command"=""}]}, {"Name"="rszvl_rng3GBSFeed", "Type"=2, "Min?"=FALSE, "Max?"=FALSE, "Entries"=[{"Name"="RSZVL_VAL_3GBS_RES_CDP", "Discrete or Min"=0.0, "Max"=0.0, "Coerced"=0.0, "Command"="'XPOW:CDP'"}, {"Name"="RSZVL_VAL_3GBS_RES_CDPABS", "Discrete or Min"=1.0, "Max"=0.0, "Coerced"=0.0, "Command"="'XPOW:CDP:ABS'"}, {"Name"="RSZVL_VAL_3GBS_RES_SUM", "Discrete or Min"=2.0, "Max"=0.0, "Coerced"=0.0, "Command"="'XTIM:CDP:ERR:SUMM'"}, {"Name"="RSZVL_VAL_3GBS_RES_CTAB", "Discrete or Min"=3.0, "Max"=0.0, "Coerced"=0.0, "Command"="'XTIM:CDP:ERR:CTAB'"}]}, {"Name"="rszvl_rng3GPPResultSumView", "Type"=2, "Min?"=FALSE, "Max?"=FALSE, "Entries"=[{"Name"="RSZVL_VAL_3GPP_RES_SUM_NORMAL", "Discrete or Min"=0.0, "Max"=0.0, "Coerced"=0.0, "Command"="NORMAL"}, {"Name"="RSZVL_VAL_3GPP_RES_SUM_EXTENDED", "Discrete or Min"=1.0, "Max"=0.0, "Coerced"=0.0, "Command"="EXTENDED"}]}, {"Name"="rszvl_rngWlanStandard", "Type"=0, "Min?"=TRUE, "Max?"=TRUE, "Entries"=[{"Name"="", "Discrete or Min"=0.0, "Max"=4.0, "Coerced"=0.0, "Command"=""}]}, {"Name"="rszvl_rngWlanPvtRPow", "Type"=2, "Min?"=FALSE, "Max?"=FALSE, "Entries"=[{"Name"="RSZVL_VAL_PVT_MEAN", "Discrete or Min"=0.0, "Max"=0.0, "Coerced"=0.0, "Command"="MEAN"}, {"Name"="RSZVL_VAL_PVT_MAX", "Discrete or Min"=1.0, "Max"=0.0, "Coerced"=0.0, "Command"="MAX"}]}, {"Name"="rszvl_rngWlanPvtSel", "Type"=2, "Min?"=FALSE, "Max?"=FALSE, "Entries"=[{"Name"="RSZVL_VAL_PVT_EDGE", "Discrete or Min"=0.0, "Max"=0.0, "Coerced"=0.0, "Command"="EDGE"}, {"Name"="RSZVL_VAL_PVT_FULL", "Discrete or Min"=1.0, "Max"=0.0, "Coerced"=0.0, "Command"="FULL"}, {"Name"="RSZVL_VAL_PVT_RISE", "Discrete or Min"=2.0, "Max"=0.0, "Coerced"=0.0, "Command"="RISE"}, {"Name"="RSZVL_VAL_PVT_FALL", "Discrete or Min"=3.0, "Max"=0.0, "Coerced"=0.0, "Command"="FALL"}]}, {"Name"="rszvl_rngWlanBurstType", "Type"=2, "Min?"=FALSE, "Max?"=FALSE, "Entries"=[{"Name"="RSZVL_VAL_WLAN_BTYP_DIRECT", "Discrete or Min"=0.0, "Max"=0.0, "Coerced"=0.0, "Command"="DIRECT"}, {"Name"="RSZVL_VAL_WLAN_BTYP_LOFDM", "Discrete or Min"=1.0, "Max"=0.0, "Coerced"=0.0, "Command"="LONG-OFDM"}, {"Name"="RSZVL_VAL_WLAN_BTYP_SOFDM", "Discrete or Min"=2.0, "Max"=0.0, "Coerced"=0.0, "Command"="SHORT-OFDM"}, {"Name"="RSZVL_VAL_WLAN_BTYP_LONG", "Discrete or Min"=3.0, "Max"=0.0, "Coerced"=0.0, "Command"="LONG"}, {"Name"="RSZVL_VAL_WLAN_BTYP_SHORT", "Discrete or Min"=4.0, "Max"=0.0, "Coerced"=0.0, "Command"="SHORT"}]}, {"Name"="rszvl_rngWlanPvtSampAver", "Type"=0, "Min?"=TRUE, "Max?"=TRUE, "Entries"=[{"Name"="", "Discrete or Min"=1.0, "Max"=399.0, "Coerced"=0.0, "Command"=""}]}, {"Name"="rszvl_rngSpecMask", "Type"=2, "Min?"=FALSE, "Max?"=FALSE, "Entries"=[{"Name"="RSZVL_VAL_SPEC_IEEE", "Discrete or Min"=0.0, "Max"=0.0, "Coerced"=0.0, "Command"="IEEE"}, {"Name"="RSZVL_VAL_SPEC_ETSI", "Discrete or Min"=1.0, "Max"=0.0, "Coerced"=0.0, "Command"="ETSI"}]}, {"Name"="rszvl_rngBurstSel", "Type"=2, "Min?"=FALSE, "Max?"=FALSE, "Entries"=[{"Name"="RSZVL_VAL_SELECTION_ALL", "Discrete or Min"=0.0, "Max"=0.0, "Coerced"=0.0, "Command"="ALL"}, {"Name"="RSZVL_VAL_SELECTION_PIL", "Discrete or Min"=1.0, "Max"=0.0, "Coerced"=0.0, "Command"="PIL"}]}, {"Name"="rszvl_rngUnitHzPct", "Type"=2, "Min?"=FALSE, "Max?"=FALSE, "Entries"=[{"Name"="RSZVL_VAL_UNIT_HZ", "Discrete or Min"=12.0, "Max"=0.0, "Coerced"=0.0, "Command"="HZ"}, {"Name"="RSZVL_VAL_UNIT_PCT", "Discrete or Min"=13.0, "Max"=0.0, "Coerced"=0.0, "Command"="PCT"}]}, {"Name"="rszvl_rngUnitDbPct", "Type"=2, "Min?"=FALSE, "Max?"=FALSE, "Entries"=[{"Name"="RSZVL_VAL_UNIT_DB", "Discrete or Min"=8.0, "Max"=0.0, "Coerced"=0.0, "Command"="DB"}, {"Name"="RSZVL_VAL_UNIT_PCT", "Discrete or Min"=13.0, "Max"=0.0, "Coerced"=0.0, "Command"="PCT"}]}, {"Name"="rszvl_rngIQSRate", "Type"=0, "Min?"=TRUE, "Max?"=TRUE, "Entries"=[{"Name"="", "Discrete or Min"=10000.0, "Max"=100000000.0, "Coerced"=0.0, "Command"=""}]}, {"Name"="rszvl_rngAutoLevelTime", "Type"=0, "Min?"=TRUE, "Max?"=TRUE, "Entries"=[{"Name"="", "Discrete or Min"=0.001, "Max"=1.0, "Coerced"=0.0, "Command"=""}]}, {"Name"="rszvl_rngPreamble", "Type"=2, "Min?"=FALSE, "Max?"=FALSE, "Entries"=[{"Name"="RSZVL_VAL_PRE_FREQ", "Discrete or Min"=0.0, "Max"=0.0, "Coerced"=0.0, "Command"="FREQ"}, {"Name"="RSZVL_VAL_PRE_PHAS", "Discrete or Min"=1.0, "Max"=0.0, "Coerced"=0.0, "Command"="PHAS"}]}, {"Name"="rszvl_rngResults", "Type"=2, "Min?"=FALSE, "Max?"=FALSE, "Entries"=[{"Name"="RSZVL_VAL_RES_FAIL", "Discrete or Min"=0.0, "Max"=0.0, "Coerced"=0.0, "Command"="FAILED"}, {"Name"="RSZVL_VAL_RES_PASS", "Discrete or Min"=1.0, "Max"=0.0, "Coerced"=0.0, "Command"="PASSED"}]}, 
